vi "Harmonics MSMT Configure External Network.vi"(8 "error in (no error)":errorcluster, 10 "Harmonic In":i8, 11 "Harmonics in":refnum<class "Harmonics.lvclass">) -> (0 "error out":errorcluster, 3 "Harmonics out":refnum<class "Harmonics.lvclass">)   [LabVIEW 2016]
uses:
  Plugins/QPA Measurement.lvlibp/QPA Measurement.lvclass
  Plugins/QPA Measurement.lvlibp/Controls/LoadPull State.ctl
  Plugins/QPA Measurement.lvlibp/Controls/External Network Parameters.ctl
  Plugins/String Database.lvlibp/String Database.lvclass
  Harmonics.lvclass
  C:/Sequence Automation/Plugins/Measurement Interface.lvlibp/Measurement Interface.lvclass
  C:/Sequence Automation/Plugins/FPF.lvlibp/Factory Plugin Framework.lvclass
  Plugins/Measurement Interface.lvlibp/Measurement Interface.lvclass
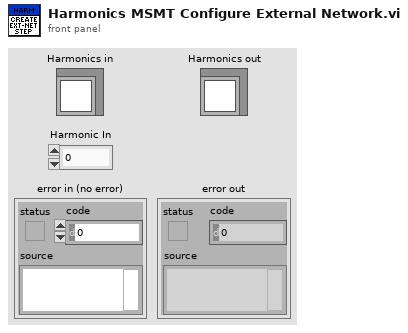
[diagram p1: front panel]
types:
  T1 = typedef "QPA Measurement.lvlibp/QPA Measurement.lvclass/LoadPull State.ctl" = enum16{"Disabled", "Coupled Path", "Uncoupled Path", "Auto"}
  T2 = typedef "QPA Measurement.lvlibp/QPA Measurement.lvclass/External Network Parameters.ctl" = cluster{"LoadPull State":T1, "SG Pin":string, "SA Pin":string, "SG Frequency":dbl, "SA Fundamental Frequency":dbl, "SG Path Name":string, "SG Sub Path Name":string, "SA Path Name":string, "SA Sub Path Name":string, "SA Measure Frequency":dbl}
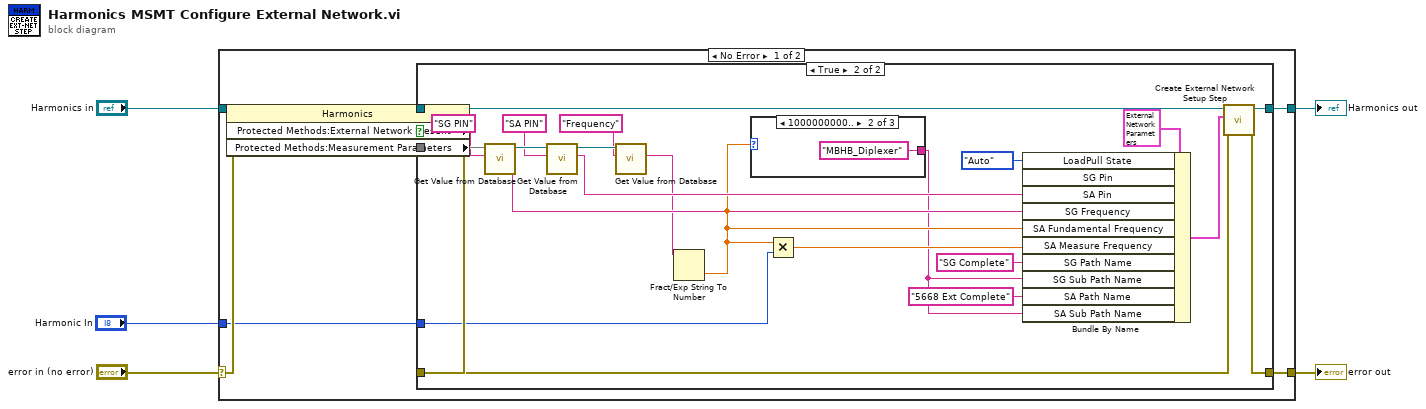
[diagram p0: block diagram]
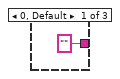
[diagram p3: hidden frame]
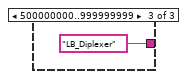
[diagram p4: hidden frame]
diagram:
  n1 = case shown="No Error" "error in (no error)" {
    selector: "error in (no error)" -> [w14 w43]
    tunnel: [w11 w43] -> w4
    tunnel: [w9 w42] -> w2
    tunnel: "Harmonics in" -> [w12 w42]
    tunnel: "Harmonic In" -> [w6 _]
    frame No Error {
      n2 = property class="Harmonics"(reference=w12, error in=w14) -> (reference out=w10:refnum<class "Harmonics.lvclass">, error out=w13:errorcluster, "Protected Methods:External Network Present"=w8, "Protected Methods:Measurement Parameters"=w7)
      n3 = case shown="True" w8 {
        tunnel: w13 -> [w15 w38]
        tunnel: [w15 w37] -> w11
        tunnel: w10 -> [w16 w36]
        tunnel: [w16 w35] -> w9
        tunnel: w7 -> [_ w33]
        tunnel: w6 -> [_ w22]
        frame False {
        }
        frame True {
          n4 = call "Get Value from Database.vi"("Entry Name"="SG PIN", "Message in"=w33) -> ("Entry Value"=w29:string, "Message out"=w31:refnum<class "String Database.lvclass">)  [unwired: 6 in, 2 out]
          n5 = call "Get Value from Database.vi"("Entry Name"="SA PIN", "Message in"=w31) -> ("Entry Value"=w28:string, "Message out"=w27:refnum<class "String Database.lvclass">)  [unwired: 6 in, 2 out]
          n6 = call "Get Value from Database.vi"("Entry Name"="Frequency", "Message in"=w27) -> ("Entry Value"=w24:string)  [unwired: 6 in, 3 out]
          n7 = Fract/Exp String To Number(string=w24) -> (number=w18:dbl)  [unwired: 3 in, 1 out]
          n8 = case shown="1000000000.." w18 {
            tunnel: ["" ("SG Path Name") "MBHB_Diplexer" ("SG Path Name") "LB_Diplexer" ("SG Path Name")] -> w17
            frame 0, Default {
            }
            frame 1000000000.. {
            }
            frame 500000000..999999999 {
            }
          }
          n9 = Multiply(x=w18, y=w22) -> (x*y=w23:dbl)
          n10 = Bundle By Name(cluster=T2 {"LoadPull State"=enum."Disabled", "SG Pin"="", "SA Pin"="", "SG Frequency"=0.0, "SA Fundamental Frequency"=0.0, "SG Path Name"="", "SG Sub Path Name"="", "SA Path Name"="", "SA Sub Path Name"="", "SA Measure Frequency"=0.0} ("External Network Parameters"), "LoadPull State"=LoadPull_State."Auto", "SG Pin"=w29, "SA Pin"=w28, "SG Frequency"=w18, "SA Fundamental Frequency"=w18, "SA Measure Frequency"=w23, "SG Path Name"="SG Complete", "SG Sub Path Name"=w17, "SA Path Name"="5668 Ext Complete", "SA Sub Path Name"=w17) -> (w21:T2)
          n11 = call "Create External Network Setup Step.vi"("error in (no error)"=w38, "External Network Parameters"=w21, "QPA Measurement in"=w36) -> ("error out"=w37:errorcluster, "QPA Measurement out"=w35:refnum<class "QPA Measurement.lvclass">)  [unwired: 7 in]
        }
      }
    }
    frame Error {
    }
  }
  "error out" <- w4
  "Harmonics out" <- w2
